vi "G#Debugger_GetEvent.vi"(5 "error in (no error)":errorcluster) -> (14 "Debugger Event":refnum<user-event>, 19 "error out":errorcluster)   [LabVIEW 2020, in "G#Debugger.lvlib"]
doc: "Returns or creates the event (if needed) used by the debugger."
uses:
  G#Debugger.lvlib
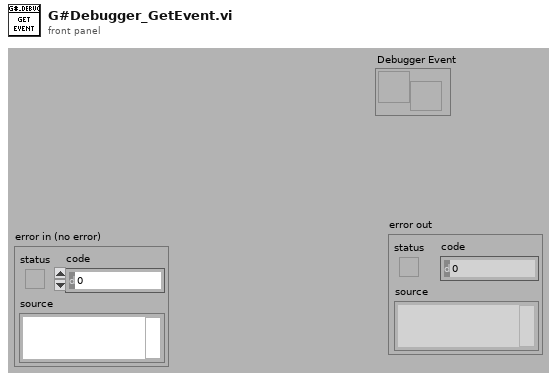
[diagram p1: front panel]
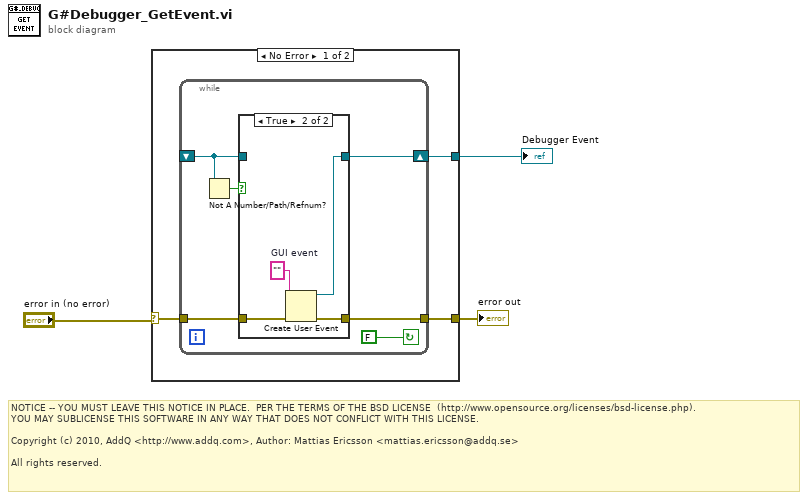
[diagram p0: block diagram]
diagram:
  # "NOTICE -- YOU MUST LEAVE THIS NOTICE IN PLACE.  PER THE TERMS OF THE BSD LICENSE  (http://www.opensource.org/licenses/bsd-license.php).\nYOU MAY SUBLICENSE THIS SOFTWARE IN ANY WAY THAT DOES NOT CONFLICT WITH THIS LICENSE.\n\nCopyright (c) 2010, AddQ <http://www.addq.com>, Author: Mattias Ericsson <mattias.ericsson@addq.se>\n\nAll rights reserved."
  n1 = case shown="No Error" "error in (no error)" {
    selector: "error in (no error)" -> [w5 w19]
    tunnel: [w6 _] -> w3
    tunnel: [w4 w19] -> w1
    frame No Error {
      n2 = while {
        tunnel: w5 -> [w11]
        tunnel: [w10] -> w4
        shift-right: [w12] -> w6
        shift-left: _ -> [w7]
        stop <- FALSE continue-if-true
        n3 = Not A Number/Path/Refnum?(number/path/refnum=w7) -> (NaN/Path/Refnum?=w8:bool)
        n4 = case shown="True" w8 {
          tunnel: [w14 w17] -> w12
          tunnel: w11 -> [w13 w16]
          tunnel: [w13 w15] -> w10
          tunnel: w7 -> [w14 _]
          frame False {
          }
          frame True {
            w18 = ""  # GUI event
            n5 = Create User Event(user event datatype=w18, error in=w16) -> (user event=w17:refnum<user-event>, error out=w15:errorcluster)
          }
        }
      }
    }
    frame Error {
    }
  }
  "Debugger Event" <- w3
  "error out" <- w1
